vi "build_read_data_query_string.vi"() -> (3 "Query String":string)   [LabVIEW 2025, in "LabJackEKG.lvlib"]
uses:
  LabJackEKG.lvlib
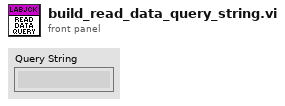
[diagram p1: front panel]
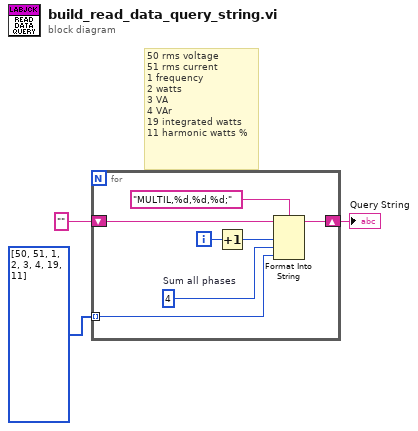
[diagram p0: block diagram]
diagram:
  # "50 rms voltage  \n51 rms current\n1 frequency  \n2 watts  \n3 VA  \n4 VAr\n19 integrated watts\n11 harmonic watts %"
  n1 = for {
    shift-right: [w8] -> w1
    shift-left: "" -> [w9]
    tunnel: i32[] [50, 51, 1, 2, 3, 4, 19, 11] -> [w7] mode=indexing
    i -> [w6]
    w4 = 4  # Sum all phases
    n2 = Increment(x=w6) -> (x+1=w5:i32)
    n3 = Format Into String(format string="MULTIL,%d,%d,%d;", initial string=w9, w5, w4, w7) -> (resulting string=w8:string)  [unwired: 1 in, 1 out]
  }
  "Query String" <- w1
